vi "RPi Main.vi"() -> ()   [LabVIEW 2021]
uses:
  Type Definitions/Data Frame.ctl
  Type Definitions/Data Frame Header.ctl
  Type Definitions/Payload Class.ctl
  Type Definitions/Device.ctl
panel:
  out "data":T1 {"CRC" format="%08x"; "Frame Header"."Options" format="%016b"; "Frame Header"."Time" format="%^<%I:%M:%S%3u %p\n%m/%d/%Y %Z>T"; "Frame Header"."Sync" format="%08x"}
  out "Recorder":variant
  out "Transmitter":variant
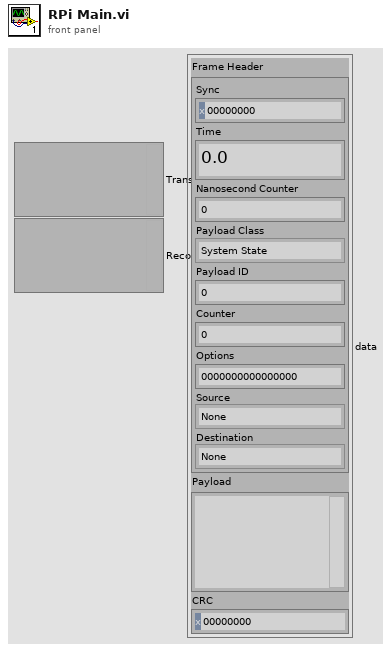
[diagram p1: front panel]
types:
  T1 = typedef "Data Frame.ctl" = cluster{"Frame Header":T2, "Payload":string, "CRC":u32}
  T2 = typedef "Data Frame Header.ctl" = cluster{"Sync":u32, "Time":dbl, "Nanosecond Counter":i64, "Payload Class":T3, "Payload ID":u16, "Counter":i32, "Options":u32, "Source":T4, "Destination":T4}
  T3 = typedef "Payload Class.ctl" = enum16{"System State", "Parameters", "Metadata", "Software Monitor", "Data", "Commands"}
  T4 = typedef "Device.ctl" = enum32{"None", "Exec", "Aux1", "Aux2", "Aux3"}
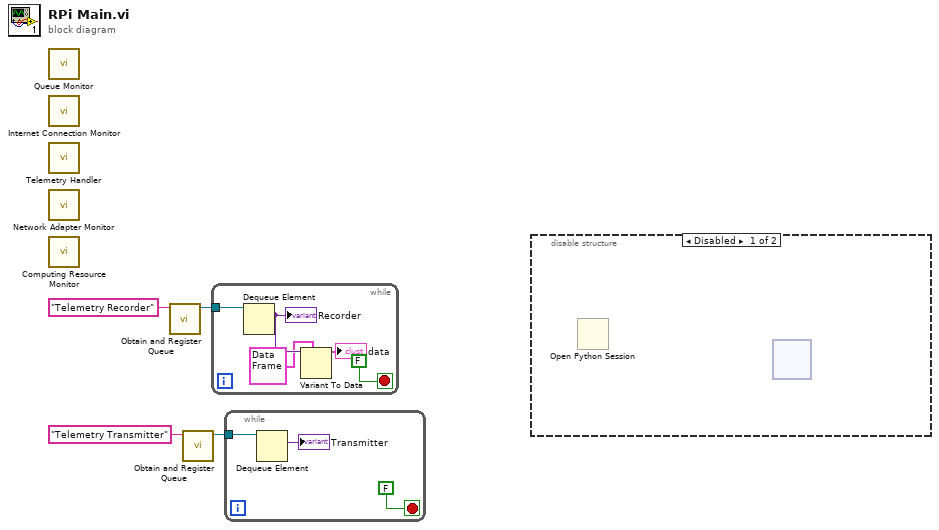
[diagram p0: block diagram]
diagram:
  n1 = call "Queue Monitor.vi"() -> ()  [unwired: 12 in]
  n2 = call "Internet Connection Monitor.vi"() -> ()  [unwired: 12 in]
  n3 = call "Telemetry Handler.vi"() -> ()  [unwired: 12 in]
  n4 = call "Network Adapter Monitor.vi"() -> ()  [unwired: 12 in]
  n5 = call "Computing Resource Monitor.vi"() -> ()  [unwired: 11 in, 1 out]
  n6 = call "Obtain and Register Queue.vi"("Queue Name (unnamed)"="Telemetry Recorder" ("name (unnamed)")) -> ("Queue Reference"=w2:refnum<queue>)  [unwired: 9 in, 1 out]
  n7 = call "Obtain and Register Queue.vi"("Queue Name (unnamed)"="Telemetry Transmitter" ("name (unnamed)")) -> ("Queue Reference"=w1:refnum<queue>)  [unwired: 9 in, 1 out]
  n8 = while {
    tunnel: w2 -> [w8]
    stop <- FALSE stop-if-true
    n9 = Dequeue Element(queue=w8) -> (element=w7:variant)  [unwired: 2 in, 3 out]
    "Recorder" <- w7
    n10 = Variant To Data(type=T1 {"Frame Header"={"Sync"=0, "Time"=0.0, "Nanosecond Counter"=0, "Payload Class"=enum."System State", "Payload ID"=0, "Counter"=0, "Options"=0, "Source"=enum."None", "Destination"=enum."None"}, "Payload"="", "CRC"=0} ("Frame"), Variant=w7) -> (data=→"data":T1)  [unwired: 1 in, 1 out]
  }
  n11 = while {
    tunnel: w1 -> [w11]
    stop <- FALSE stop-if-true
    n12 = Dequeue Element(queue=w11) -> (element=→"Transmitter":variant)  [unwired: 2 in, 3 out]
  }
  n13 = disable-structure shown="Disabled" {
    frame Disabled {
      n14 = Open Python Session() -> ()  [unwired: 3 in, 2 out]
      n15 = node() -> ()  [unwired: 6 in, 4 out]
    }
    frame Enabled {
    }
  }
